vi "Insert Row.vi"(7 "SheetName":string, 8 "error in":errorcluster, 9 "Row Index":i32, 10 "New Row":refnum<k24>, 11 "SpreadsheetDocument in":refnum<k24>) -> (0 "error out":errorcluster, 3 "SpreadsheetDocument out":refnum<k24>)   [LabVIEW 2021, in "Open Xml.lvlib"]
uses:
  Open Xml.lvlib
  D:/git/Open-Xml-LabVIEW/dll/DocumentFormat.OpenXml.dll
  dll/DocumentFormat.OpenXml.dll
  D:/git/Open-Xml-LabVIEW/dll/DocumentFormat.OpenXml.Framework.dll
  dll/DocumentFormat.OpenXml.Framework.dll
  D:/git/Open-Xml-LabVIEW/dll/OpenXmlGenericsWrapper.dll
  dll/OpenXmlGenericsWrapper.dll
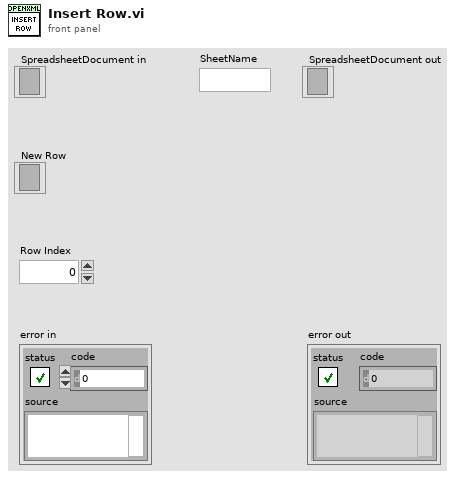
[diagram p1: front panel]
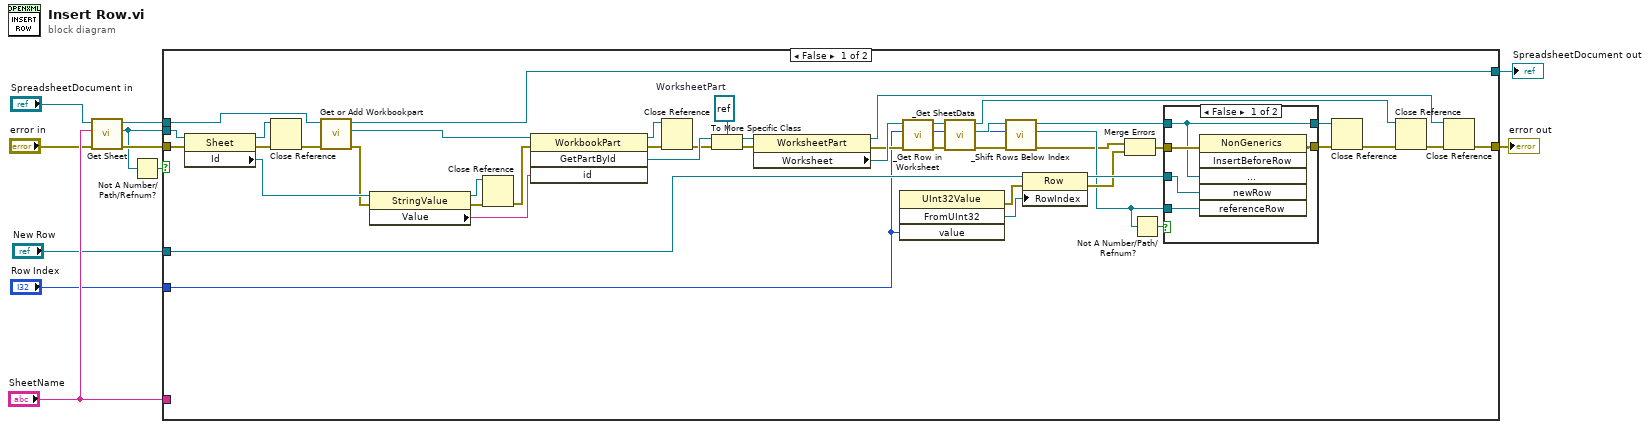
[diagram p0: block diagram]
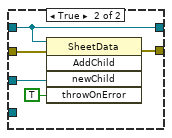
[diagram p2: hidden frame]
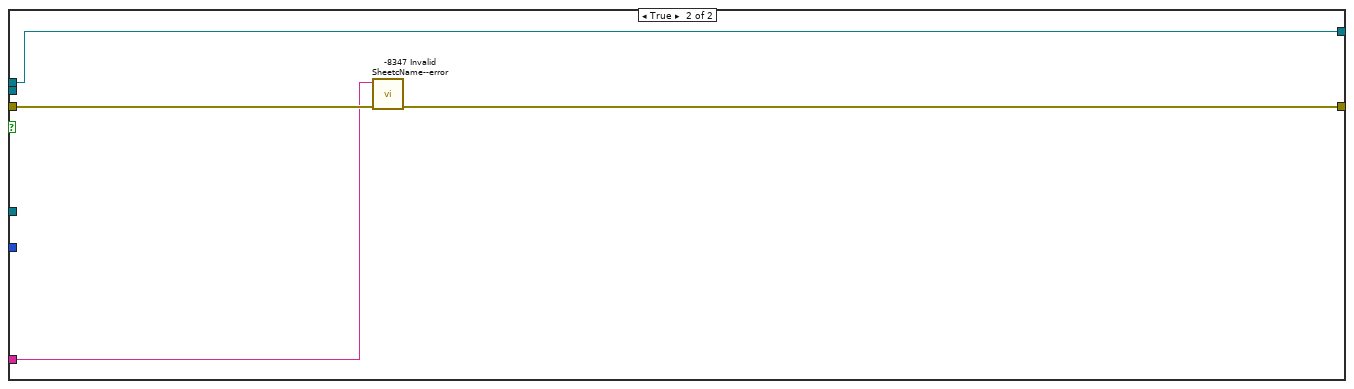
[diagram p3: hidden frame]
diagram:
  n1 = call "Get Sheet.vi"("error in"="error in", "SheetName"="SheetName", "SpreadsheetDoc in"="SpreadsheetDocument in") -> ("error out"=w5:errorcluster, "Sheet"=w2:refnum<k24>, "SpreadsheetDoc out"=w4:refnum<k24>)  [unwired: 6 in]
  n2 = Not A Number/Path/Refnum?(number/path/refnum=w2) -> (NaN/Path/Refnum?=w6:bool)
  n3 = case shown="False" w6 {
    tunnel: [w44 w66] -> w11
    tunnel: [w38 w68] -> w10
    tunnel: "SheetName" -> [_ w67]
    tunnel: w5 -> [w52 w69]
    tunnel: w4 -> [w55 w66]
    tunnel: "Row Index" -> [w20 _]
    tunnel: w2 -> [w53 _]
    tunnel: "New Row" -> [w24 _]
    frame False {
      w45 = refnum<k24> refnum  # WorksheetPart
      n4 = property class="Sheet"(reference=w53, error in=w52) -> (reference out=w35:refnum<k24>, error out=w51:errorcluster, "Id"=w50:refnum<k24>)
      n5 = Close Reference(reference=w35, error in (no error)=w51) -> (error out=w36:errorcluster)
      n6 = call "Get or Add Workbookpart.vi"("error in"=w36, "SpreadsheetDocument"=w55) -> ("error out"=w43:errorcluster, "WorkbookPart"=w54:refnum<k24>, "SpreadsheetDocument out"=w44:refnum<k24>)  [unwired: 7 in]
      n7 = property class="StringValue"(reference=w50, error in=w43) -> (reference out=w48:refnum<k24>, error out=w26:errorcluster, "Value"=w49:string)
      n8 = Close Reference(reference=w48, error in (no error)=w26) -> (error out=w25:errorcluster)
      n9 = invoke class="WorkbookPart" method="GetPartById"(reference=w54, error in=w25, "id"=w49) -> (reference out=w33:refnum<k24>, error out=w47:errorcluster, "GetPartById"=w46:refnum<k24>)  [unwired: 1 in, 1 out]
      n10 = Close Reference(reference=w33, error in (no error)=w47) -> (error out=w34:errorcluster)
      n11 = To More Specific Class(target class=w45, reference=w46, error in=w34) -> (specific class reference=w41:refnum<k24>, error out=w42:errorcluster)
      n12 = property class="WorksheetPart"(reference=w41, error in=w42) -> (reference out=w37:refnum<k24>, error out=w28:errorcluster, "Worksheet"=w39:refnum<k24>)
      n13 = invoke class="UInt32Value" method="FromUInt32"("value"=w20) -> (error out=w19:errorcluster, "FromUInt32"=w21:refnum<k24>)  [unwired: 3 in, 2 out]
      n14 = call "_Get Row in Worksheet.vi"("error in"=w28, "RowIndex"=w20) -> ("error out"=w29:errorcluster)  [unwired: 7 in, 2 out]
      n15 = call "_Get SheetData.vi"("error in"=w29, "Worksheet in"=w39) -> ("error out"=w27:errorcluster, "SheetData"=w30:refnum<k24>, "Worksheet out"=w32:refnum<k24>)  [unwired: 7 in]
      n16 = call "_Shift Rows Below Index.vi"("error in"=w27, "Row Index"=w20, "SheetData in"=w30) -> ("error out"=w14:errorcluster, "Reference Row"=w17:refnum<k24>, "SheetData out"=w13:refnum<k24>)  [unwired: 6 in]
      n17 = property class="Row"(reference=w24, error in=w19, "RowIndex"=w21) -> (reference out=w22:refnum<k24>, error out=w18:errorcluster)
      n18 = Merge Errors(w14, w18) -> (w15:errorcluster)
      n19 = Not A Number/Path/Refnum?(number/path/refnum=w17) -> (NaN/Path/Refnum?=w16:bool)
      n20 = case shown="False" w16 {
        tunnel: [w60 w64] -> w31
        tunnel: w17 -> [w59 _]
        tunnel: w22 -> [w58 w62]
        tunnel: w15 -> [w57 w65]
        tunnel: w13 -> [w56 w61]
        tunnel: [w56 w61] -> w12
        frame False {
          n21 = invoke class="NonGenerics" method="InsertBeforeRow"(error in=w57, "sheetData"=w56, "newRow"=w58, "referenceRow"=w59) -> (error out=w60:errorcluster)  [unwired: 2 in, 5 out]
        }
        frame True {
          n22 = invoke class="SheetData" method="AddChild"(reference=w61, error in=w65, "newChild"=w62, "throwOnError"=TRUE) -> (error out=w64:errorcluster)  [unwired: 1 in, 4 out]
        }
      }
      n23 = Close Reference(reference=w12, error in (no error)=w31) -> (error out=w23:errorcluster)
      n24 = Close Reference(reference=w32, error in (no error)=w23) -> (error out=w40:errorcluster)
      n25 = Close Reference(reference=w37, error in (no error)=w40) -> (error out=w38:errorcluster)
    }
    frame True {
      n26 = call "-8347 Invalid SheetcName--error.vi"("error in"=w69, "Argument"=w67) -> ("error out"=w68:errorcluster)  [unwired: 9 in]
    }
  }
  "error out" <- w10
  "SpreadsheetDocument out" <- w11
